vi "myTimer.vi"(8 "error in (no error)":errorcluster, 10 "TimeTarget":dbl, 11 "Reset?":bool) -> (0 "error out":errorcluster, 2 "TimeElapsed?":bool, 3 "ElpasedTime":dbl)   [LabVIEW 2020]
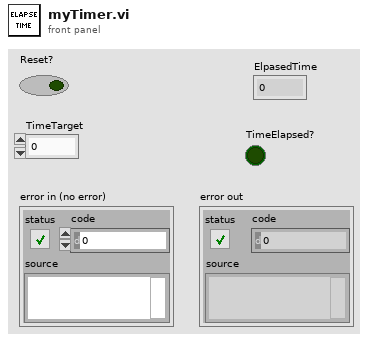
[diagram p1: front panel]
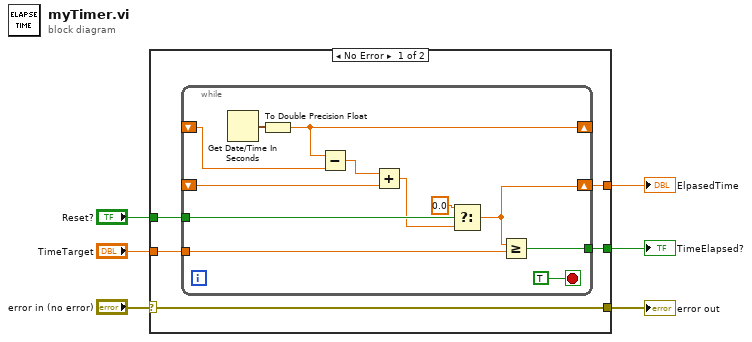
[diagram p0: block diagram]
diagram:
  n1 = case shown="No Error" "error in (no error)" {
    selector: "error in (no error)" -> [w10 w24]
    tunnel: [w11 _] -> w6
    tunnel: [w10 w24] -> w4
    tunnel: "Reset?" -> [w9 _]
    tunnel: "TimeTarget" -> [w8 _]
    tunnel: [w7 _] -> w1
    frame No Error {
      n2 = while {
        shift-right: [w22] -> _
        shift-left: _ -> [w21]
        shift-right: [w14] -> w11
        shift-left: _ -> [w18]
        tunnel: w9 -> [w17]
        tunnel: w8 -> [w13]
        tunnel: [w12] -> w7
        stop <- TRUE stop-if-true
        n3 = Get Date/Time In Seconds() -> (seconds since 1Jan1904=w23:timestamp)
        n4 = To Double Precision Float(number=w23) -> (double precision float=w22:dbl)
        n5 = Subtract(x=w22, y=w21) -> (x-y=w19:dbl)
        n6 = Add(x=w19, y=w18) -> (x+y=w15:dbl)
        n7 = Select(t=0.0, s=w17, f=w15) -> (s? t:f=w14:dbl)
        n8 = Greater Or Equal?(x=w14, y=w13) -> (x >= y?=w12:bool)
      }
    }
    frame Error {
    }
  }
  "error out" <- w4
  "ElpasedTime" <- w6
  "TimeElapsed?" <- w1
